vi "ChannelTypetoClass.vi"(11 "channel name":string) -> (3 "string":string)   [LabVIEW 2015, in "Group.lvclass"]
doc: "Copyright 2017 National Instruments Corporation\n\nLicensed under the Apache License, Version 2.0 (the \"License\"); you may not use this file except in compliance with the License. You may obtain a copy of the License at http://www.apache.org/licenses/LICENSE-2.0\nUnless required by applicable law or agreed to in writing, software distributed under the License is distributed on an \"AS IS\" BASIS, WITHOUT WARRANTIES OR CONDITIONS OF ANY KIND, either express or implied. See the License for the specific language governing permissions and limitations under the License."
uses:
  Group.lvclass
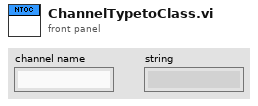
[diagram p1: front panel]
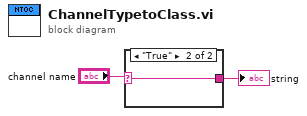
[diagram p0: block diagram]
diagram:
  n1 = case shown="\"True\"" "channel name" {
    selector: "channel name" -> [_ w3]
    tunnel: [_ w3] -> w2
    frame "False", Default {
    }
    frame "True" {
    }
  }
  "string" <- w2
